vi "Menu.vi"() -> ()   [LabVIEW 2020, in "SwipeMenu.lvclass"]
uses:
  SwipeMenu.lvclass
  SwipeMenu.lvclass/SwipeMenu.ctl
  Demo Buttons/Test Button.ctl
  Demo Buttons/About Button.ctl
  Demo Buttons/Dismiss Popup.ctl
  Demo Buttons/QSI Button.ctl
  Demo Buttons/Checkbox Demo Button.ctl
  Demo Buttons/Dialogs Demo Button.ctl
  Demo Buttons/Example SubMenu Button.ctl
  Demo Buttons/Filter Clicks.ctl
  Demo Buttons/Listbox Demo Button.ctl
  Demo Buttons/OSK Demo Button.ctl
  Demo Buttons/Scrollbar Demo Button.ctl
  Demo Buttons/String Scrollbar Demo Button.ctl
  Demo Buttons/Swipe Scroll Button.ctl
  Demo Buttons/Swipe Select Button.ctl
  Menu Cluster.ctl
panel:
  in  "Menu Cluster":T1
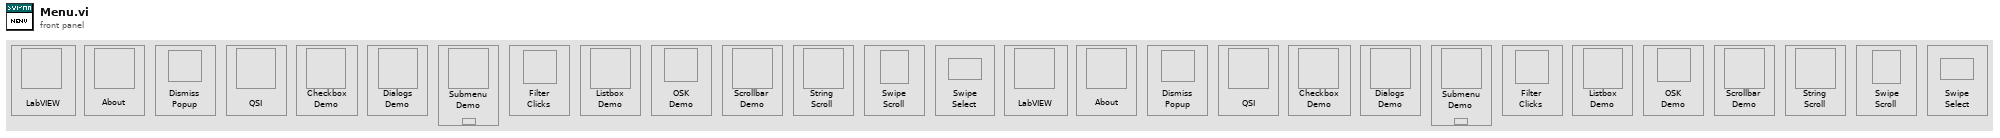
[diagram p1: front panel]
types:
  T1 = typedef "SwipeMenu.lvclass/Menu Cluster.ctl" = cluster{"LabVIEW":T2, "About":T3, "Dismiss Popup":T4, "QSI":T5, "Checkboxes Demo":T6, "Dialog Demo":T7, "Submenu Demo":T8, "Filter Clicks":T9, "Listboxes Demo":T10, "OSK Demo":T11, "Scrollbar Demo":T12, "String Demo":T13, "Swipe Scroll":T14, "Swipe Select":T15, "LabVIEW 2":T2, "About 2":T3, "Dismiss Popup 2":T4, "QSI 2":T5, "Checkboxes Demo 2":T6, "Dialog Demo 2":T7, "Submenu Demo 2":T8, "Filter Clicks 2":T9, "Listboxes Demo 2":T10, "OSK Demo 2":T11, "Scrollbar Demo 2":T12, "String Demo 2":T13, "Swipe Scroll 2":T14, "Swipe Select 2":T15}
  T2 = typedef "Test Button.ctl" = bool
  T3 = typedef "About Button.ctl" = bool
  T4 = typedef "Dismiss Popup.ctl" = bool
  T5 = typedef "QSI Button.ctl" = bool
  T6 = typedef "Checkbox Demo Button.ctl" = bool
  T7 = typedef "Dialogs Demo Button.ctl" = bool
  T8 = typedef "Example SubMenu Button.ctl" = bool
  T9 = typedef "Filter Clicks.ctl" = bool
  T10 = typedef "Listbox Demo Button.ctl" = bool
  T11 = typedef "OSK Demo Button.ctl" = bool
  T12 = typedef "Scrollbar Demo Button.ctl" = bool
  T13 = typedef "String Scrollbar Demo Button.ctl" = bool
  T14 = typedef "Swipe Scroll Button.ctl" = bool
  T15 = typedef "Swipe Select Button.ctl" = bool
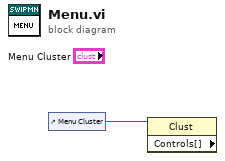
[diagram p0: block diagram]
diagram:
  n1 = control-ref of="Menu Cluster"() -> (w1:refnum<vi>)
  n2 = property class="Clust" props=["Controls[]"](reference=w1) -> ()  [unwired: 1 in, 3 out]
